vi "Test Driver Message Loop.vi"(8 "error in (no error)":errorcluster) -> (0 "error out":errorcluster)   [LabVIEW 2020, in "Test Driver.lvlib"]
doc: "Message loop for handling messages pertaining to the acquisition of data from the hardware."
uses:
  Test Driver.lvlib
  support/PCT FGV CMD.ctl
  Acquisition State.ctl
  Test Driver Configuration.ctl
  support/Message Queue/Message Cluster.ctl
  System Preset.ctl
  Test Type.ctl
  Popup/Popup Dialog States.ctl
  Motion/AM Configuration.ctl
  support/Message Queue/Enqueue Message (Single).vi
  support/REF Single  Name to ref convert.vi
  <vilib>/Utility/error.llb/Error Cluster From Error Code.vi
  <vilib>/ErrorRing/Error Ring.xnode
  support/Message Queue/Message Queue.lvlib
  Popup/Popup Dialog.lvlib
  Motion/Motion.lvlib
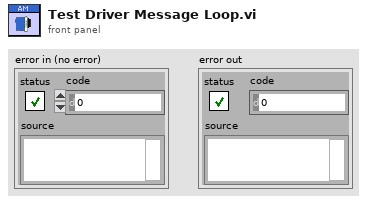
[diagram p1: front panel]
types:
  T1 = typedef "PCT FGV CMD.ctl" = enum16{"INIT", "GET", "SET"}
  T2 = typedef "PCT Data REFs.ctl" = cluster{"PLC AI Notifier":refnum<notifier>, "PS Data Queue":refnum<queue>, "BTN Queue":refnum<queue>, "PLC DI notifier":refnum<notifier>, "Timer notifier":refnum<notifier>, "DMM PS":refnum<notifier>, "DMM Gages":refnum<notifier>, "XYZ notifier":refnum<notifier>, "Test Notifier":refnum<notifier>, "Scanner notifier":refnum<notifier>, "OPC Notifier":refnum<notifier>, "HIDEN queue":refnum<queue>}
  T3 = typedef "Message Queue.lvlib/All Message Queues.ctl" = cluster{"UI":refnum<queue>, "Logging":refnum<queue>, "LOG":refnum<queue>, "ALARM":refnum<queue>, "Test":refnum<queue>, "Answer":refnum<queue>, "PLC":refnum<queue>, "DB":refnum<queue>, "Report":refnum<queue>, "OPC":refnum<queue>, "Procedure":refnum<queue>, "PalmSens":refnum<queue>, "SYS 7000 Reader":refnum<queue>, "SWITCH":refnum<queue>, "MOTOR":refnum<queue>, "MOTION":refnum<queue>, "HIDEN":refnum<queue>, "VALVE":refnum<queue>, "MFC":refnum<queue>, "PUMP IN":refnum<queue>, "PUMP OUT":refnum<queue>}
  T4 = typedef "Test Driver.lvlib/Test Driver Configuration.ctl" = cluster{"current Step":i32, "Wait":dbl, "Next Step":string, "Writer Queue":refnum<queue>, "Reset":bool, "SEQ Time":i32, "General Reset":bool, "Cycles":i32, "Status":bool[], "Ready":bool[], "Backward":bool, "Current SP":dbl[], "System Preset":T5, "Test Type":T6, "Sample Count":i32, "Local Queues":cluster{"Cycles queue":refnum<queue>, "Step queue":refnum<queue>, "RES Queue":refnum<queue>, "Clean queue":refnum<queue>, "PS Scan queue":refnum<queue>}, "current Clean":i32, "PS Measure Plan":u16[]}
  T5 = typedef "System Preset.ctl" = cluster{"Test Configuration":cluster{"Cycles":i32, "Z Up":dbl, "SP List":dbl[][], "Operator":string, "Point Delay":i32, "Z Up 2":dbl, "Cleaning In":dbl, "Cleaning Out":dbl, "Cleaning Cycles":i32}, "Test_Start_date":string}
  T6 = typedef "Test Driver.lvlib/Test Type.ctl" = enum16{"Calibration", "Test"}
  T7 = typedef "Test Driver.lvlib/Acquisition State.ctl" = enum16{"Idle", "Initialized"}
  T8 = typedef "Popup Dialog.lvlib/Popup Dialog States.ctl" = enum32{"Complete", "Failed", "Preparing", "Stopping", "Error", "Saved", "Saving", "Closing"}
  T9 = cluster{"Writer Queue":refnum<queue>, "Timeout":dbl[], "Status":bool[]}
  T10 = typedef "Motion.lvlib/AM Configuration.ctl" = cluster{"Wait":dbl, "Next Step":string, "Writer Queue":refnum<queue>, "Reset":bool, "Target":dbl[]}
  T11 = typedef "Message Queue.lvlib/Message Cluster.ctl" = cluster{"Message":string, "Message Data":variant}
  T12 = typedef "MeasurementResults.ctl" = T13[]
  T13 = typedef "LiveCurveResult.ctl" = cluster{"X Label":string, "Y Label":string, "Name":string, "Index":i16, "Curve Values":cluster{"Values":cluster{"X Value":dbl, "Y Value":dbl}[], "Index":i16}}
  T14 = cluster{"whole match":string, "Results":T12, "Measurements":dbl[]}
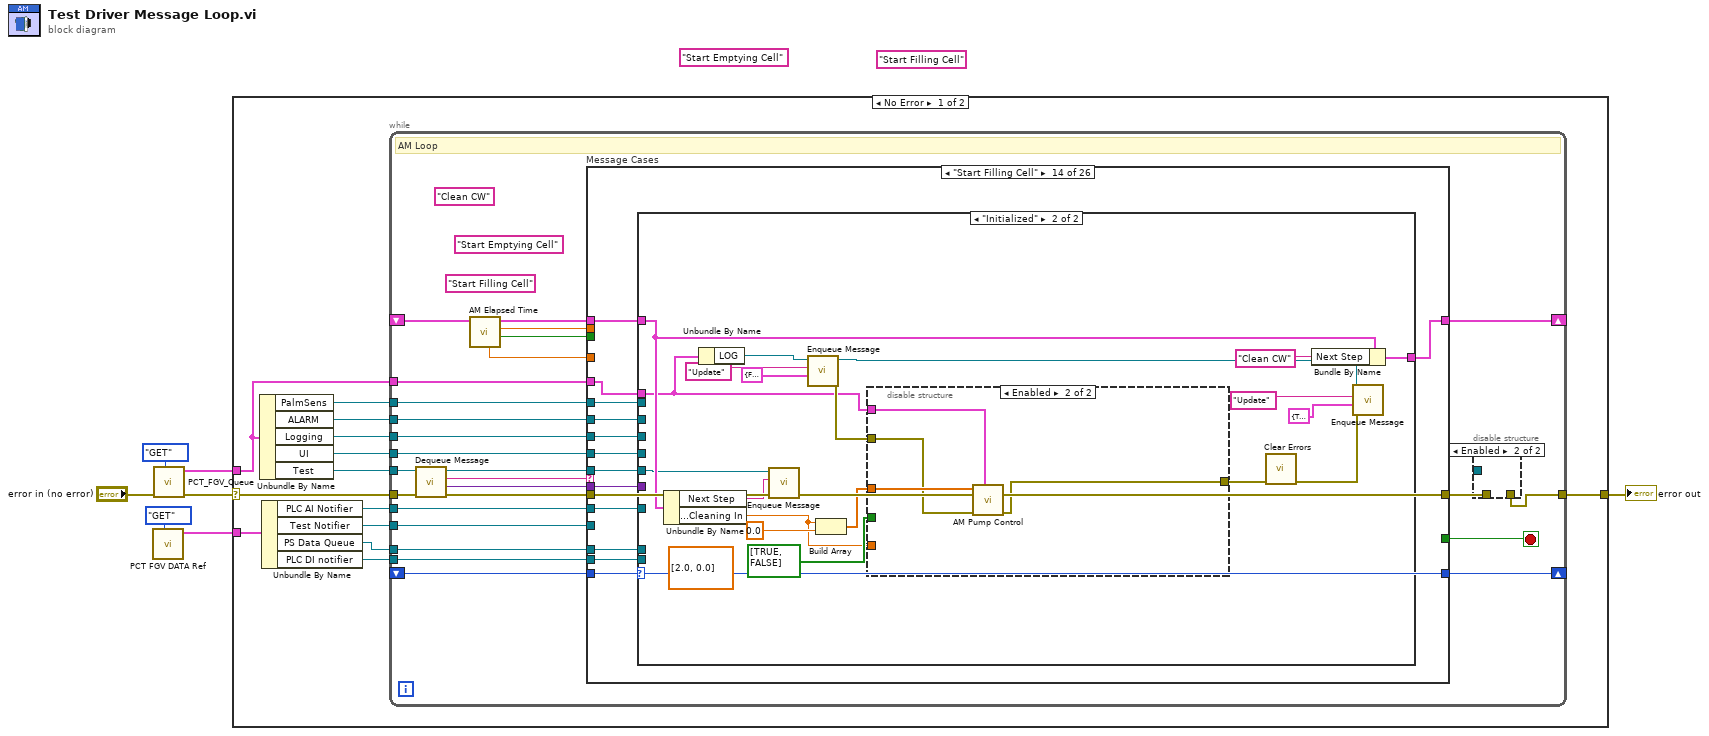
[diagram p0: block diagram]
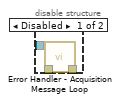
[diagram p2: hidden frame]
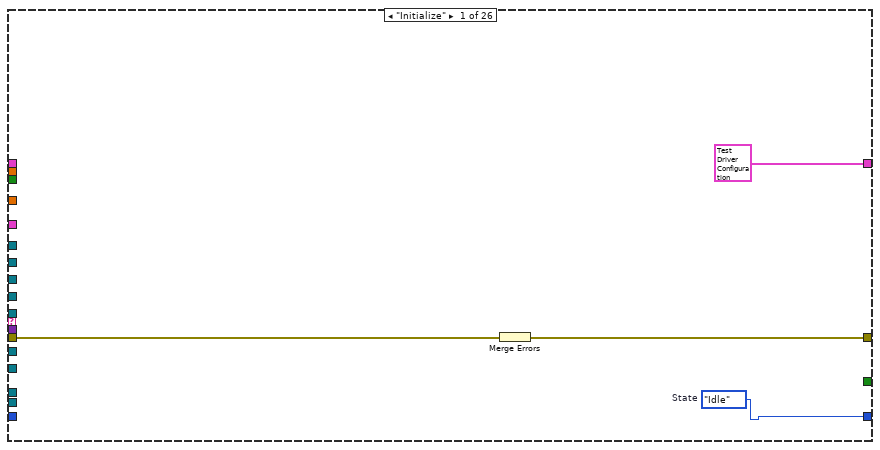
[diagram p3: hidden frame]
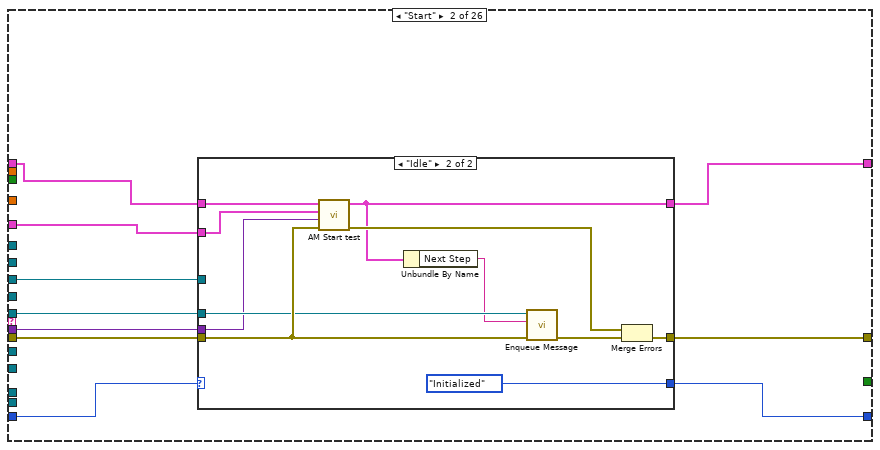
[diagram p4: hidden frame]
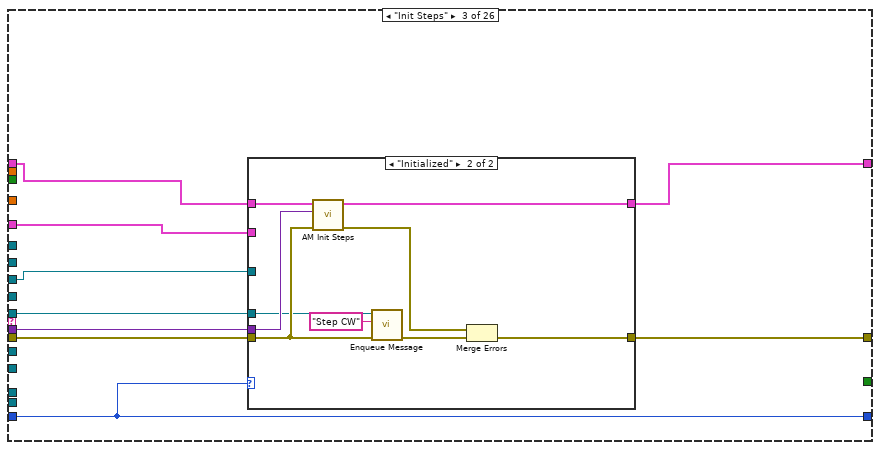
[diagram p6: hidden frame]
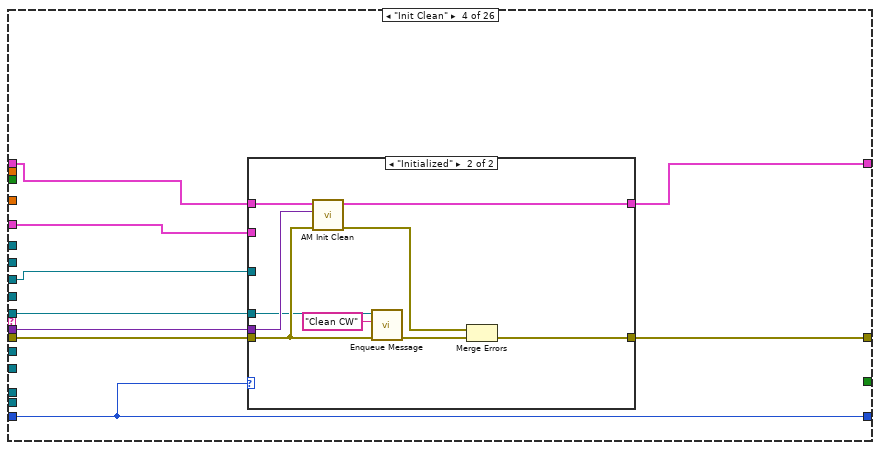
[diagram p8: hidden frame]
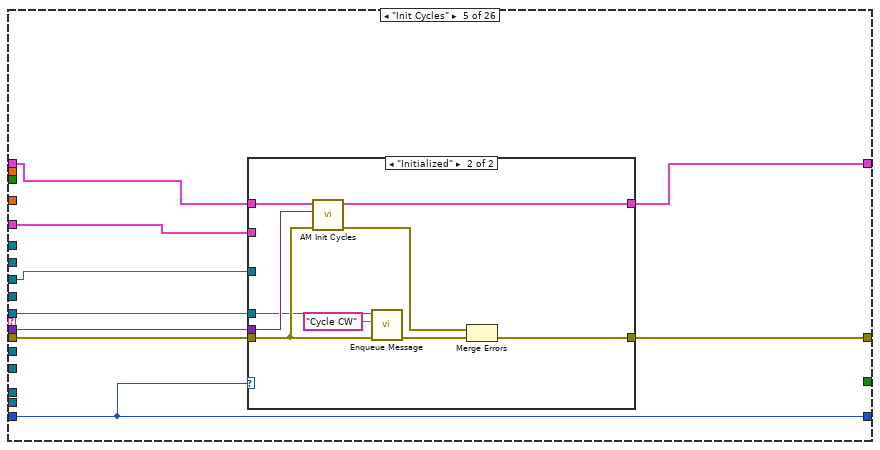
[diagram p10: hidden frame]
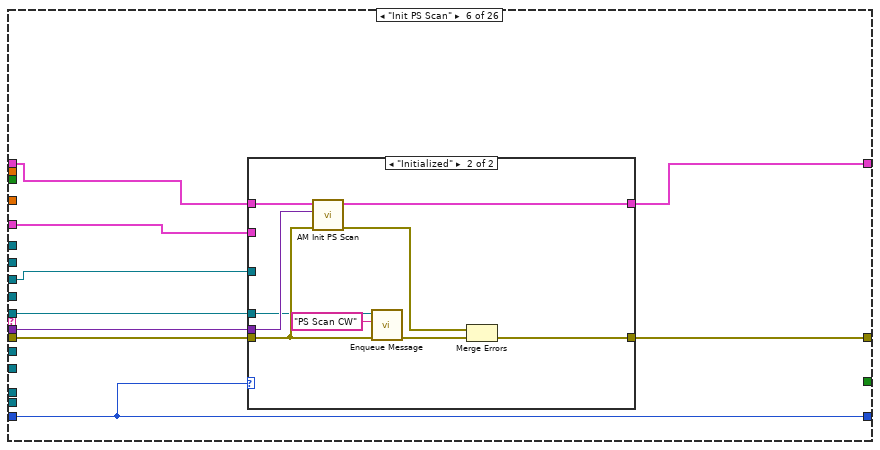
[diagram p12: hidden frame]
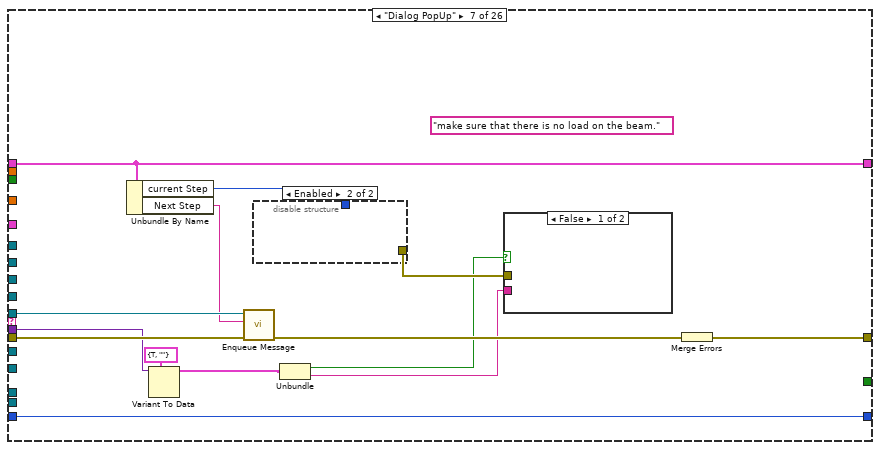
[diagram p14: hidden frame]
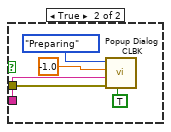
[diagram p15: hidden frame]
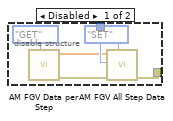
[diagram p16: hidden frame]
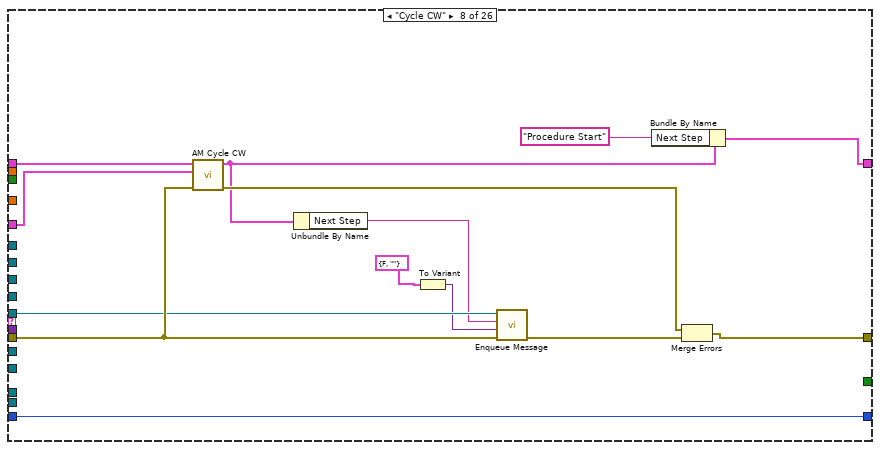
[diagram p17: hidden frame]
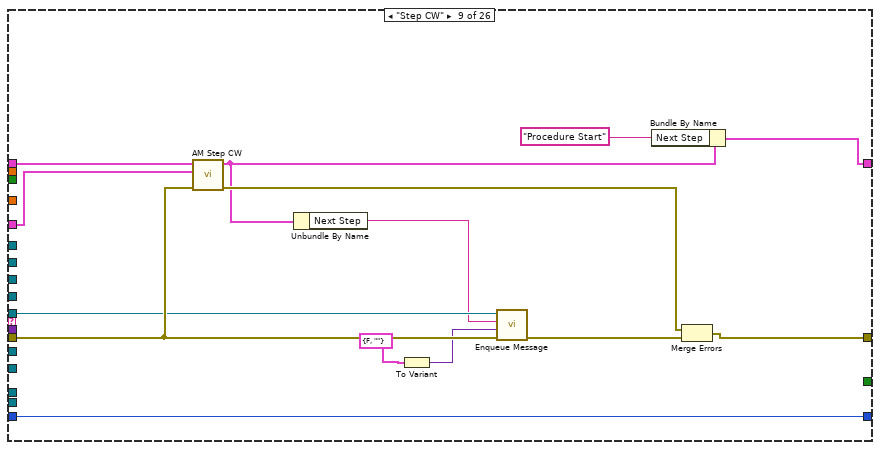
[diagram p18: hidden frame]
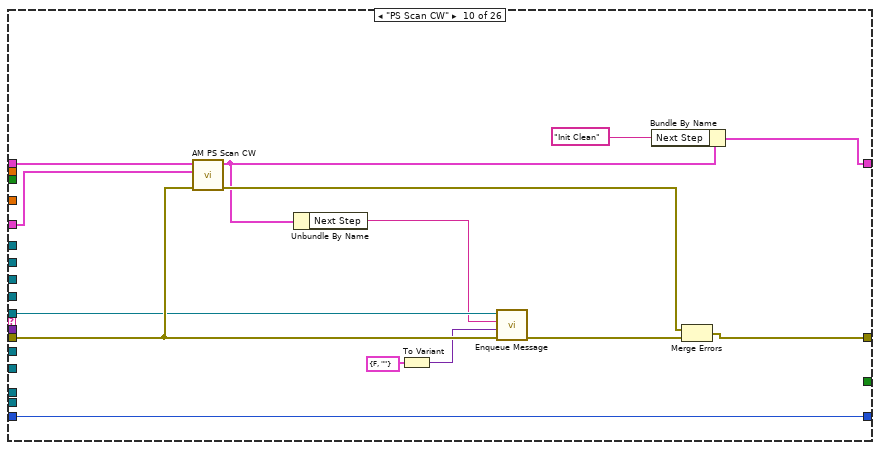
[diagram p19: hidden frame]
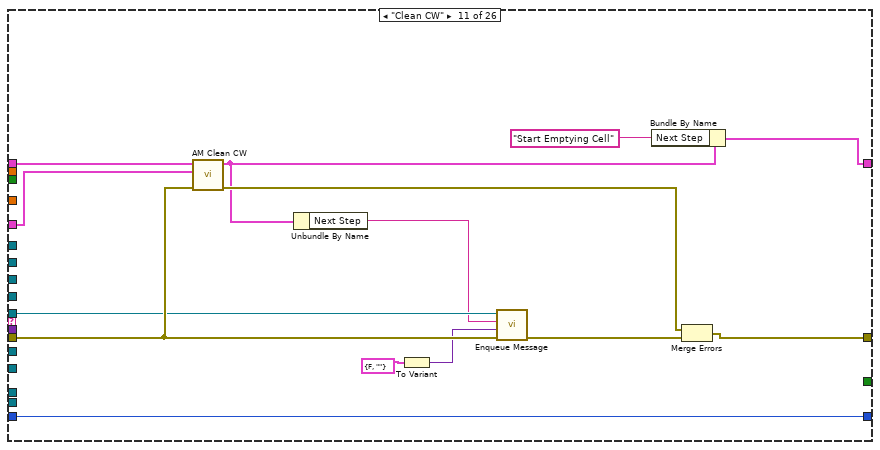
[diagram p20: hidden frame]
diagram:
  (unwired) "Start Filling Cell"
  (unwired) "Start Emptying Cell"
  n1 = call "PCT FGV DATA Ref.vi"("CMD"=PCT_FGV_CMD."GET") -> ("Data REF"=w1:T2)  [unwired: 9 in, 1 out]
  n2 = call "PCT_FGV_Queue.vi"("CMD"=PCT_FGV_CMD."GET", "error in (no error)"="error in (no error)") -> ("error out"=w4:errorcluster, "Message Queues out"=w3:T3)  [unwired: 8 in]
  n3 = case shown="No Error" w4 {
    selector: w4 -> [w18 w653]
    tunnel: w3 -> [w16 _]
    tunnel: [w19 w653] -> w7
    tunnel: w1 -> [w15 _]
    frame No Error {
      n4 = Unbundle By Name(w16) -> ("PalmSens"=w10:refnum<queue>, "ALARM"=w12:refnum<queue>, "Logging"=w13:refnum<queue>, "UI"=w17:refnum<queue>, "Test"=w20:refnum<queue>)
      n5 = Unbundle By Name(w15) -> ("PLC AI Notifier"=w9:refnum<notifier>, "Test Notifier"=w14:refnum<notifier>, "PS Data Queue"=w11:refnum<queue>, "PLC DI notifier"=w8:refnum<notifier>)
      n6 = while {
        tunnel: w20 -> [w39]
        shift-right: [w45] -> _
        shift-left: _ -> [w46]
        tunnel: w17 -> [w33]
        shift-right: [w37] -> _
        shift-left: _ -> [w38]
        tunnel: w16 -> [w29]
        tunnel: w18 -> [w43]
        tunnel: [w36] -> w19
        tunnel: w14 -> [w27]
        tunnel: w13 -> [w26]
        tunnel: w12 -> [w25]
        tunnel: w11 -> [w24]
        tunnel: w10 -> [w23]
        tunnel: w9 -> [w22]
        tunnel: w8 -> [w21]
        stop <- w44 stop-if-true
        (unwired) "Clean CW" ("Message")
        (unwired) "Start Emptying Cell"
        (unwired) "Start Filling Cell" ("Message")
        # "AM Loop"
        n7 = call "Dequeue Message.vi"("error in (no error)"=w43, "Message Queue"=w39) -> ("error out"=w42:errorcluster, "Message Data"=w40:variant, "Message"=w41:string, "dup Message Queue"=w34:refnum<queue>)  [unwired: 6 in]
        n8 = call "AM Elapsed Time.vi"("AM Refs in"=w46) -> ("Time has Elapsed"=w31:bool, "Start Elapsed Time"=w28:dbl, "AM Refs out"=w32:T4, "Elapsed Time (s)"=w30:dbl)  [unwired: 7 in]
        n9 = case "Message Cases" shown="\"Start Filling Cell\"" w41 {
          selector: w41 -> [_ _ _ _ _ _ _ _ _ _ _ w240 _ _ _ _ _ _ _ _ _ _ _ _ _ w642]
          tunnel: w34 -> [_ w60 w83 w103 w123 w143 w168 w190 w204 w218 w232 w247 w263 w319 w377 w436 w481 _ w574 w603 w608 w612 _ _ w636 _]
          tunnel: w42 -> [w52 w61 w84 w104 w124 w144 w169 w191 w205 w219 w233 w248 w265 w321 w379 w438 w500 w537 w575 w604 w609 w616 w624 w628 w638 _]
          tunnel: [w53 w63 w86 w106 w126 w146 w166 w193 w207 w221 w235 w250 w265 w321 w379 w438 w500 w537 w575 w604 w609 w615 w623 w634 w640 w643] -> w35
          tunnel: w32 -> [_ w62 w85 w105 w125 w145 w167 w195 w209 w223 w237 w246 w260 w316 w374 w433 w493 w533 w551 w590 w610 w617 w621 w630 w639 w645]
          tunnel: [T4 {"current Step"=0, "Wait"=0.0, "Next Step"="", "Writer Queue"=refnum, "Reset"=FALSE, "SEQ Time"=0, "General Reset"=FALSE, "Cycles"=0, "Status"=[], "Ready"=[], "Backward"=FALSE, "Current SP"=[], "System Preset"={"Test Configuration"={"Cycles"=0, "Z Up"=0.0, "SP List"=[], "Operator"="", "Point Delay"=0, "Z Up 2"=0.0, "Cleaning In"=0.0, "Cleaning Out"=0.0, "Cleaning Cycles"=0}, "Test_Start_date"=""}, "Test Type"=enum."Calibration", "Sample Count"=0, "Local Queues"={"Cycles queue"=refnum, "Step queue"=refnum, "RES Queue"=refnum, "Clean queue"=refnum, "PS Scan queue"=refnum}, "current Clean"=0, "PS Measure Plan"=[]} ("Data Cluster") w59 w82 w102 w122 w142 w167 w186 w200 w214 w228 w242 w264 w320 w378 w437 w499 w536 w571 w599 w610 w618 w621 w629 w639 w645] -> w45
          tunnel: [_ _ _ _ _ _ _ _ _ _ _ _ _ _ _ _ _ _ _ _ _ _ _ _ TRUE _] -> w44
          tunnel: w40 -> [_ w56 w81 w101 w121 w141 w162 _ _ _ _ w239 w261 w317 w375 w434 _ _ _ _ _ w614 w622 w633 _ _]
          tunnel: w33 -> [_ _ _ _ _ _ _ _ _ _ _ _ w258 w314 w372 w431 _ _ _ _ _ _ _ _ _ _]
          tunnel: w38 -> [_ w57 w79 w99 w119 w139 w171 w196 w210 w224 w238 w251 w252 w308 w366 w425 w501 w538 _ _ _ w619 w625 w627 _ w644]
          tunnel: [w51 w58 w79 w99 w119 w139 w171 w196 w210 w224 w238 w251 w252 w308 w366 w425 w501 w538 Acquisition_State."Idle" ("Acquisition State") Acquisition_State."Idle" ("Acquisition State") Acquisition_State."Idle" ("Acquisition State") w619 w625 w627 Acquisition_State."Idle" ("Acquisition State") w644] -> w37
          tunnel: w31 -> [_ _ _ _ _ _ _ _ _ _ _ w241 _ _ _ _ _ _ _ _ _ _ _ _ _ _]
          tunnel: w30 -> [_ _ _ _ _ _ _ _ _ _ _ _ _ _ _ _ _ _ _ _ _ _ _ _ _ _]
          tunnel: w29 -> [_ w55 w80 w100 w120 w140 _ w194 w208 w222 w236 _ w262 w318 w376 w435 w491 w534 w560 w591 _ w613 _ _ _ _]
          tunnel: w28 -> [_ _ _ _ _ _ _ _ _ _ _ _ _ _ _ _ _ _ _ _ _ _ _ _ _ _]
          tunnel: w27 -> [_ _ _ _ _ _ _ _ _ _ _ _ _ _ _ _ _ w532 _ _ _ _ _ _ _ _]
          tunnel: w26 -> [_ w54 w78 w98 w118 w138 _ _ _ _ _ _ w255 w311 w369 w428 _ _ _ w582 _ _ _ _ _ _]
          tunnel: w25 -> [_ _ _ _ _ _ _ _ _ _ _ _ w259 w315 w373 w432 _ _ _ _ _ _ _ _ _ _]
          tunnel: w24 -> [_ _ _ _ _ _ _ _ _ _ _ _ w257 w313 w371 w430 _ _ _ _ _ _ _ _ _ _]
          tunnel: w23 -> [_ _ _ _ _ _ _ _ _ _ _ _ w256 w312 w370 w429 _ _ _ _ _ _ _ _ _ _]
          tunnel: w22 -> [_ _ _ _ _ _ _ _ _ _ _ _ w254 w310 w368 w427 _ _ _ _ _ _ _ _ _ _]
          tunnel: w21 -> [_ _ _ _ _ _ _ _ _ _ _ _ w253 w309 w367 w426 _ _ _ _ _ _ _ _ _ _]
          frame "Initialize" {
            w51 = Acquisition_State."Idle"  # State
            # "Initialize  - Initialize is currently a no-op.  The hardware initialization takes place in the 'Start' message."
            n10 = Merge Errors(w52) -> (w53:errorcluster)
          }
          frame "Start" {
            # "Start - Configure and start the acquisition."
            n11 = case shown="\"Idle\"" w57 {
              selector: w57 -> [w64 _]
              tunnel: [w65 w77] -> w63
              tunnel: w62 -> [w66 w76]
              tunnel: w61 -> [w65 w73]
              tunnel: w60 -> [_ w71]
              tunnel: [w66 w68] -> w59
              tunnel: [w64 Acquisition_State."Initialized" ("Acquisition State")] -> w58
              tunnel: w56 -> [_ w69]
              tunnel: w55 -> [_ w70]
              tunnel: w54 -> [_ _]
              frame "Initialized" {
                # "The system is already acquiring. Ignore the \"Start\" message."
              }
              frame "Idle" {
                # "If the system is idle, start the acquisition."
                n12 = call "AM Start test.vi"("error in (no error)"=w73, "Variant"=w69, "Message Queues in"=w70, "Hardware Resources in"=w76) -> ("error out"=w75:errorcluster, "Hardware Resources out"=w68:T4)  [unwired: 6 in]
                n13 = Unbundle By Name(w68) -> ("Next Step"=w67:string)
                n14 = call-poly "Enqueue Message.vi"("error in (no error)"=w73, "Message"=w67, "Message Queue"=w71) -> ("error out"=w72:errorcluster)  [unwired: 7 in, 1 out]
                n15 = Merge Errors(w75, w72) -> (w77:errorcluster)
              }
            }
          }
          frame "Init Steps" {
            # "Start - Configure and start the acquisition."
            n16 = case shown="\"Initialized\"" w79 {
              tunnel: [w87 w97] -> w86
              tunnel: w85 -> [w88 w96]
              tunnel: w84 -> [w87 w93]
              tunnel: w83 -> [_ w91]
              tunnel: [w88 w89] -> w82
              tunnel: w81 -> [_ w94]
              tunnel: w80 -> [_ _]
              tunnel: w78 -> [_ _]
              frame "Idle" {
                # "The system is already acquiring. Ignore the \"Start\" message."
              }
              frame "Initialized" {
                # "If the system is idle, start the acquisition."
                n17 = call "AM Init Steps.vi"("error in (no error)"=w93, "Message Data"=w94, "Hardware Resources in"=w96) -> ("error out"=w95:errorcluster, "Hardware Resources out"=w89:T4)  [unwired: 7 in]
                n18 = call-poly "Enqueue Message.vi"("error in (no error)"=w93, "Message"="Step CW", "Message Queue"=w91) -> ("error out"=w92:errorcluster)  [unwired: 7 in, 1 out]
                n19 = Merge Errors(w95, w92) -> (w97:errorcluster)
              }
            }
          }
          frame "Init Clean" {
            # "Start - Configure and start the acquisition."
            n20 = case shown="\"Initialized\"" w99 {
              tunnel: [w107 w117] -> w106
              tunnel: w105 -> [w108 w116]
              tunnel: w104 -> [w107 w113]
              tunnel: w103 -> [_ w111]
              tunnel: [w108 w109] -> w102
              tunnel: w101 -> [_ w114]
              tunnel: w100 -> [_ _]
              tunnel: w98 -> [_ _]
              frame "Idle" {
                # "The system is already acquiring. Ignore the \"Start\" message."
              }
              frame "Initialized" {
                # "If the system is idle, start the acquisition."
                n21 = call "AM Init Clean.vi"("error in (no error)"=w113, "Message Data"=w114, "Hardware Resources in"=w116) -> ("error out"=w115:errorcluster, "Hardware Resources out"=w109:T4)  [unwired: 7 in]
                n22 = call-poly "Enqueue Message.vi"("error in (no error)"=w113, "Message"="Clean CW", "Message Queue"=w111) -> ("error out"=w112:errorcluster)  [unwired: 7 in, 1 out]
                n23 = Merge Errors(w115, w112) -> (w117:errorcluster)
              }
            }
          }
          frame "Init Cycles" {
            # "Start - Configure and start the acquisition."
            n24 = case shown="\"Initialized\"" w119 {
              tunnel: [w127 w137] -> w126
              tunnel: w125 -> [w128 w136]
              tunnel: w124 -> [w127 w133]
              tunnel: w123 -> [_ w131]
              tunnel: [w128 w129] -> w122
              tunnel: w121 -> [_ w134]
              tunnel: w120 -> [_ _]
              tunnel: w118 -> [_ _]
              frame "Idle" {
                # "The system is already acquiring. Ignore the \"Start\" message."
              }
              frame "Initialized" {
                # "If the system is idle, start the acquisition."
                n25 = call "AM Init Cycles.vi"("error in (no error)"=w133, "Message Data"=w134, "Hardware Resources in"=w136) -> ("error out"=w135:errorcluster, "Hardware Resources out"=w129:T4)  [unwired: 7 in]
                n26 = call-poly "Enqueue Message.vi"("error in (no error)"=w133, "Message"="Cycle CW", "Message Queue"=w131) -> ("error out"=w132:errorcluster)  [unwired: 7 in, 1 out]
                n27 = Merge Errors(w135, w132) -> (w137:errorcluster)
              }
            }
          }
          frame "Init PS Scan" {
            # "Start - Configure and start the acquisition."
            n28 = case shown="\"Initialized\"" w139 {
              tunnel: [w147 w157] -> w146
              tunnel: w145 -> [w148 w156]
              tunnel: w144 -> [w147 w153]
              tunnel: w143 -> [_ w151]
              tunnel: [w148 w149] -> w142
              tunnel: w141 -> [_ w154]
              tunnel: w140 -> [_ _]
              tunnel: w138 -> [_ _]
              frame "Idle" {
                # "The system is already acquiring. Ignore the \"Start\" message."
              }
              frame "Initialized" {
                # "If the system is idle, start the acquisition."
                n29 = call "AM Init PS Scan.vi"("error in (no error)"=w153, "Message Data"=w154, "Hardware Resources in"=w156) -> ("error out"=w155:errorcluster, "Hardware Resources out"=w149:T4)  [unwired: 7 in]
                n30 = call-poly "Enqueue Message.vi"("error in (no error)"=w153, "Message"="PS Scan CW", "Message Queue"=w151) -> ("error out"=w152:errorcluster)  [unwired: 7 in, 1 out]
                n31 = Merge Errors(w155, w152) -> (w157:errorcluster)
              }
            }
          }
          frame "Dialog PopUp" {
            (unwired) "make sure that there is no load on the beam." ("String")
            # "Start - Configure and start the acquisition."
            n32 = Unbundle By Name(w167) -> ("current Step"=w165:i32, "Next Step"=w164:string)
            n33 = Variant To Data(type=cluster{"Show":bool, "Message":string} {"Show"=TRUE, "Message"=""}, Variant=w162) -> (data=w160:cluster{"Show":bool, "Message":string})  [unwired: 1 in, 1 out]
            n34 = call-poly "Enqueue Message.vi"("error in (no error)"=w169, "Message"=w164, "Message Queue"=w168) -> ("error out"=w170:errorcluster)  [unwired: 7 in, 1 out]
            n35 = disable-structure shown="Enabled" {
              disable-tunnel: w165 -> [w182 _]
              disable-tunnel: [w178 _] -> w163
              frame Disabled {
                n36 = call "AM FGV Data per Step.vi"("CMD"=PCT_FGV_CMD."GET") -> ("error out"=w179:errorcluster, "All Data out"=w177:dbl[])  [unwired: 9 in]
                n37 = call "AM FGV All Step Data.vi"("CMD"=PCT_FGV_CMD."SET", "error in (no error)"=w179, "current Step"=w182, "Proc Data in"=w177) -> ("error out"=w178:errorcluster)  [unwired: 6 in, 1 out]
              }
              frame Enabled {
              }
            }
            n38 = Unbundle(w160) -> ("Show"=w159:bool, "Message"=w158:string)
            n39 = case shown="False" w159 {
              tunnel: w163 -> [_ w175]
              tunnel: w158 -> [_ w173]
              frame False {
              }
              frame True {
                n40 = call "Popup Dialog CLBK.vi"("show"=TRUE, "error in"=w175, "String"=w173, "Delay (5sec)"=-1.0, "Tab Control"=Popup_Dialog_States."Preparing") -> ()  [unwired: 4 in, 3 out]
              }
            }
            n41 = Merge Errors(w170) -> (w166:errorcluster)
          }
          frame "Cycle CW" {
            # "Start - Configure and start the acquisition."
            n42 = call "AM Cycle CW.vi"("error in (no error)"=w191, "Message Queues in"=w194, "Data Cluster"=w195) -> ("error out"=w188:errorcluster, "Data Cluster out"=w187:T4)  [unwired: 7 in]
            n43 = Unbundle By Name(w187) -> ("Next Step"=w189:string)
            n44 = To Variant(anything=cluster{"Show":bool, "Message":string} {"Show"=FALSE, "Message"=""}) -> (Variant=w183:variant)
            n45 = call-poly "Enqueue Message.vi"("error in (no error)"=w191, "Message Data"=w183, "Message"=w189, "Message Queue"=w190) -> ("error out"=w192:errorcluster)  [unwired: 6 in, 1 out]
            n46 = Bundle By Name(cluster=w187, "Next Step"="Procedure Start" ("Message")) -> (w186:T4)
            n47 = Merge Errors(w188, w192) -> (w193:errorcluster)
          }
          frame "Step CW" {
            # "Start - Configure and start the acquisition."
            n48 = call "AM Step CW.vi"("error in (no error)"=w205, "Message Queues in"=w208, "Data Cluster"=w209) -> ("error out"=w202:errorcluster, "Data Cluster out"=w201:T4)  [unwired: 7 in]
            n49 = Unbundle By Name(w201) -> ("Next Step"=w203:string)
            n50 = To Variant(anything=cluster{"Show":bool, "Message":string} {"Show"=FALSE, "Message"=""}) -> (Variant=w197:variant)
            n51 = call-poly "Enqueue Message.vi"("error in (no error)"=w205, "Message Data"=w197, "Message"=w203, "Message Queue"=w204) -> ("error out"=w206:errorcluster)  [unwired: 6 in, 1 out]
            n52 = Bundle By Name(cluster=w201, "Next Step"="Procedure Start" ("Message")) -> (w200:T4)
            n53 = Merge Errors(w202, w206) -> (w207:errorcluster)
          }
          frame "PS Scan CW" {
            # "Start - Configure and start the acquisition."
            n54 = call "AM PS Scan CW.vi"("error in (no error)"=w219, "Message Queues in"=w222, "Data Cluster"=w223) -> ("error out"=w216:errorcluster, "Data Cluster out"=w215:T4)  [unwired: 7 in]
            n55 = Unbundle By Name(w215) -> ("Next Step"=w217:string)
            n56 = To Variant(anything=cluster{"Show":bool, "Message":string} {"Show"=FALSE, "Message"=""}) -> (Variant=w211:variant)
            n57 = call-poly "Enqueue Message.vi"("error in (no error)"=w219, "Message Data"=w211, "Message"=w217, "Message Queue"=w218) -> ("error out"=w220:errorcluster)  [unwired: 6 in, 1 out]
            n58 = Bundle By Name(cluster=w215, "Next Step"="Init Clean" ("Message")) -> (w214:T4)
            n59 = Merge Errors(w216, w220) -> (w221:errorcluster)
          }
          frame "Clean CW" {
            # "Start - Configure and start the acquisition."
            n60 = call "AM Clean CW.vi"("error in (no error)"=w233, "Message Queues in"=w236, "Data Cluster"=w237) -> ("error out"=w230:errorcluster, "Data Cluster out"=w229:T4)  [unwired: 7 in]
            n61 = Unbundle By Name(w229) -> ("Next Step"=w231:string)
            n62 = To Variant(anything=cluster{"Show":bool, "Message":string} {"Show"=FALSE, "Message"=""}) -> (Variant=w226:variant)
            n63 = call-poly "Enqueue Message.vi"("error in (no error)"=w233, "Message Data"=w226, "Message"=w231, "Message Queue"=w232) -> ("error out"=w234:errorcluster)  [unwired: 6 in, 1 out]
            n64 = Bundle By Name(cluster=w229, "Next Step"="Start Emptying Cell") -> (w228:T4)
            n65 = Merge Errors(w230, w234) -> (w235:errorcluster)
          }
          frame "Wait" {
            # "Start - Configure and start the acquisition."
            n66 = Unbundle By Name(w246) -> ("Next Step"=w245:string)
            n67 = Wait Until Next ms Multiple(millisecond multiple=u32 200) -> ()  [unwired: 1 out]
            n68 = Select(t=w245, s=w241, f=w240) -> (s? t:f=w244:string)
            n69 = Bundle By Name(cluster=w246, "Reset"=w241) -> (w242:T4)
            n70 = call-poly "Enqueue Message.vi"("error in (no error)"=w248, "Message Data"=w239, "Message"=w244, "Message Queue"=w247) -> ("error out"=w249:errorcluster)  [unwired: 6 in, 1 out]
            n71 = Merge Errors(w249) -> (w250:errorcluster)
          }
          frame "Procedure Response" {
            # "Start - Configure and start the acquisition."
            n72 = case shown="\"Initialized\"" w252 {
              tunnel: [w266 w303] -> w264
              tunnel: w263 -> [_ w301]
              tunnel: w262 -> [_ w293]
              tunnel: w261 -> [_ _]
              tunnel: w260 -> [w266 w292]
              tunnel: w259 -> [_ w291]
              tunnel: w258 -> [_ w282]
              tunnel: w257 -> [_ _]
              tunnel: w256 -> [_ _]
              tunnel: w255 -> [_ _]
              tunnel: w254 -> [_ _]
              tunnel: w253 -> [_ _]
              frame "Idle", Default {
              }
              frame "Initialized" {
                (unwired) "PS Scan"
                w272 = PCT_FGV_CMD."SET" ("CMD")
                n73 = call-poly "Enqueue Message.vi"("Message"="Stop", "Message Queue"=w291) -> ()  [unwired: 8 in, 2 out]
                n74 = Unbundle By Name(w292) -> ("Current SP"=w283:dbl[], "current Step"=w268:i32, "Cycles"=w271:i32)
                n75 = call-poly "Enqueue Message.vi"("Message"="Start Filling Cell", "Message Queue"=w301) -> ()  [unwired: 8 in, 2 out]
                n76 = Build Array (concatenate)(w283, w268) -> (w276:dbl[])
                n77 = for {
                  tunnel: string[] ["X%0.1f ", "Y%0.1f "] ("format string") -> [w307] mode=indexing
                  tunnel: w283 -> [w306] mode=indexing
                  shift-right: [w305] -> w288
                  shift-left: "" -> [w304]
                  n78 = Format Into String(format string=w307, initial string=w304, w306) -> (resulting string=w305:string)  [unwired: 1 in, 1 out]
                }
                n79 = call "FGV Parameters.vi"("CMD"=w272, "input"=w268, "Key"="Step") -> ("error out"=w269:errorcluster)  [unwired: 6 in, 2 out]
                n80 = call "FGV Parameters.vi"("CMD"=w272, "error in (no error)"=w269, "input"=w271, "Key"="Cycle") -> ()  [unwired: 5 in, 3 out]
                n81 = Format Into String(format string="Movement to %s has finished", w288) -> (resulting string=w295:string)  [unwired: 2 in, 1 out]
                n82 = Unbundle By Name(w293) -> ("LOG"=w294:refnum<queue>)
                n83 = Reverse 1D Array(array=w276) -> (reversed array=w274:dbl[])
                n84 = Bundle By Name(cluster=cluster{"Replace":bool, "String":string} {"Replace"=FALSE, "String"="Procedure was started"}, "String"=w295) -> (w296:cluster{"Replace":bool, "String":string})
                n85 = Number To Fractional String(number=w274, precision (6)=i16 1) -> (F-format string=w275:string[])  [unwired: 2 in]
                n86 = call "Bundle CMD Queue Cluster.vi"("Message Data"=w276, "Message"="Update Procedure" ("Type CMD")) -> ("Message Cluster"=w286:T11)  [unwired: 9 in]
                n87 = call "Bundle CMD Queue Cluster.vi"("Message Data"=w275, "Message"="Update RES Table" ("Type CMD")) -> ("Message Cluster"=w280:T11)  [unwired: 9 in]
                n88 = call-poly "Enqueue Message.vi"("Message Data"=w286, "Message"="Update Status" ("Main CMD"), "Message Queue"=w282) -> ("dup Message Queue"=w278:refnum<queue>)  [unwired: 7 in, 1 out]
                n89 = call-poly "Enqueue Message.vi"("Message Data"=w296, "Message"="Update" ("Main CMD"), "Message Queue"=w294) -> ()  [unwired: 7 in, 2 out]
                n90 = Bundle By Name(cluster=w292, "Next Step"="Init PS Scan") -> (w303:T4)
                n91 = call-poly "Enqueue Message.vi"("Priority Message? (F)"=TRUE, "Message Data"=w280, "Message"="Update Status", "Message Queue"=w278) -> ()  [unwired: 6 in, 2 out]
              }
            }
          }
          frame "Start Filling Cell" {
            # "Start - Configure and start the acquisition."
            n92 = case shown="\"Initialized\"" w308 {
              tunnel: [w322 w341] -> w320
              tunnel: w319 -> [_ w336]
              tunnel: w318 -> [_ w323]
              tunnel: w317 -> [_ _]
              tunnel: w316 -> [w322 w338]
              tunnel: w315 -> [_ _]
              tunnel: w314 -> [_ _]
              tunnel: w313 -> [_ _]
              tunnel: w312 -> [_ _]
              tunnel: w311 -> [_ _]
              tunnel: w310 -> [_ _]
              tunnel: w309 -> [_ _]
              frame "Idle", Default {
              }
              frame "Initialized" {
                (unwired) dbl[] [2.0, 0.0] ("Timeout")
                n93 = Unbundle By Name(w338) -> ("Next Step"=w328:string, "System Preset.Test Configuration.Cleaning In"=w324:dbl)
                n94 = Unbundle By Name(w323) -> ("LOG"=w331:refnum<queue>)
                n95 = call-poly "Enqueue Message.vi"("Message"=w328, "Message Queue"=w336) -> ()  [unwired: 8 in, 2 out]
                n96 = call-poly "Enqueue Message.vi"("Message Data"=cluster{"Replace":bool, "String":string} {"Replace"=FALSE, "String"="Cell Filling->START"}, "Message"="Update" ("Main CMD"), "Message Queue"=w331) -> ("error out"=w329:errorcluster, "dup Message Queue"=w330:refnum<queue>)  [unwired: 7 in]
                n97 = Build Array(w324, 0.0 ("Timeout")) -> (w325:dbl[])
                n98 = disable-structure shown="Enabled" {
                  disable-tunnel: w323 -> [w355 w362]
                  disable-tunnel: bool[] [TRUE, FALSE] ("Status") -> [w352 _]
                  disable-tunnel: [w347 w364] -> w335
                  disable-tunnel: w329 -> [w346 w363]
                  disable-tunnel: w325 -> [w344 w365]
                  disable-tunnel: w324 -> [w343 _]
                  frame Disabled {
                    n99 = call "Obtain Message Queue.vi"() -> ("Message Queue"=w351:refnum<queue>)  [unwired: 10 in, 1 out]
                    n100 = Bundle By Name(cluster=T9 {"Writer Queue"=refnum, "Timeout"=[], "Status"=[]}, "Writer Queue"=w351, "Timeout"=w344, "Status"=w352) -> (w353:T9)
                    n101 = call-poly "Enqueue Message.vi"("error in (no error)"=w346, "Message Data"=w353, "Message"="Start", "Message Queue"=w355) -> ("error out"=w350:errorcluster)  [unwired: 6 in, 1 out]
                    n102 = Multiply(x=w343, y=2000.0) -> (x*y=w348:dbl)
                    n103 = for {
                      N: 2 -> [_]
                      tunnel: w348 -> [w358]
                      shift-right: [w357] -> w342
                      shift-left: w351 -> [w361]
                      tunnel: w350 -> [w360]
                      tunnel: [w359] -> w347
                      n104 = Dequeue Element(queue=w361, timeout in ms (-1)=w358, error in (no error)=w360) -> (queue out=w357:refnum<queue>, error out=w359:errorcluster)  [unwired: 2 out]
                    }
                    n105 = Release Queue(queue=w342) -> ()  [unwired: 2 in, 3 out]
                  }
                  frame Enabled {
                    n106 = call "AM Pump Control.vi"("input cluster"=w362, "error in (no error)"=w363, "Times"=w365) -> ("error out"=w364:errorcluster)  [unwired: 8 in]
                  }
                }
                n107 = call <vilib>:"Clear Errors.vi"("error in (no error)"=w335) -> ("error out"=w334:errorcluster)  [unwired: 5 in, 1 out]
                n108 = Bundle By Name(cluster=w338, "Next Step"="Clean CW" ("Message")) -> (w341:T4)
                n109 = call-poly "Enqueue Message.vi"("error in (no error)"=w334, "Message Data"=cluster{"Replace":bool, "String":string} {"Replace"=TRUE, "String"="Cell Filling->DONE"}, "Message"="Update" ("Main CMD"), "Message Queue"=w330) -> ()  [unwired: 6 in, 2 out]
              }
            }
          }
          frame "Start Emptying Cell" {
            # "Start - Configure and start the acquisition."
            n110 = case shown="\"Initialized\"" w366 {
              tunnel: [w380 w399] -> w378
              tunnel: w377 -> [_ w395]
              tunnel: w376 -> [_ w381]
              tunnel: w375 -> [_ _]
              tunnel: w374 -> [w380 w387]
              tunnel: w373 -> [_ _]
              tunnel: w372 -> [_ _]
              tunnel: w371 -> [_ _]
              tunnel: w370 -> [_ _]
              tunnel: w369 -> [_ _]
              tunnel: w368 -> [_ _]
              tunnel: w367 -> [_ _]
              frame "Idle", Default {
              }
              frame "Initialized" {
                (unwired) dbl[] [0.0, 5.0] ("Timeout")
                n111 = Unbundle By Name(w381) -> ("LOG"=w390:refnum<queue>)
                n112 = Unbundle By Name(w387) -> ("Next Step"=w386:string, "System Preset.Test Configuration.Cleaning Out"=w383:dbl)
                n113 = call-poly "Enqueue Message.vi"("Message"=w386, "Message Queue"=w395) -> ()  [unwired: 8 in, 2 out]
                n114 = call-poly "Enqueue Message.vi"("Message Data"=cluster{"Replace":bool, "String":string} {"Replace"=FALSE, "String"="Cell Emptying>START"}, "Message"="Update" ("Main CMD"), "Message Queue"=w390) -> ("error out"=w388:errorcluster, "dup Message Queue"=w389:refnum<queue>)  [unwired: 7 in]
                n115 = Build Array(0.0 ("Timeout"), w383) -> (w382:dbl[])
                n116 = disable-structure shown="Enabled" {
                  disable-tunnel: w381 -> [w414 w422]
                  disable-tunnel: bool[] [FALSE, TRUE] ("Status") -> [w411 _]
                  disable-tunnel: [w405 w423] -> w394
                  disable-tunnel: w388 -> [w404 w421]
                  disable-tunnel: w382 -> [w401 w424]
                  frame Disabled {
                    n117 = call "Obtain Message Queue.vi"() -> ("Message Queue"=w410:refnum<queue>)  [unwired: 10 in, 1 out]
                    n118 = Bundle By Name(cluster=T9 {"Writer Queue"=refnum, "Timeout"=[], "Status"=[]}, "Writer Queue"=w410, "Timeout"=w401, "Status"=w411) -> (w412:T9)
                    n119 = Index Array(array=w401, index=1) -> (element=w408:dbl)
                    n120 = call-poly "Enqueue Message.vi"("error in (no error)"=w404, "Message Data"=w412, "Message"="Start", "Message Queue"=w414) -> ("error out"=w409:errorcluster)  [unwired: 6 in, 1 out]
                    n121 = Multiply(x=w408, y=2000.0) -> (x*y=w406:dbl)
                    n122 = for {
                      N: 2 -> [_]
                      tunnel: w406 -> [w418]
                      shift-right: [w416] -> w400
                      shift-left: w410 -> [w420]
                      tunnel: w409 -> [w419]
                      tunnel: [w417] -> w405
                      n123 = Dequeue Element(queue=w420, timeout in ms (-1)=w418, error in (no error)=w419) -> (queue out=w416:refnum<queue>, error out=w417:errorcluster)  [unwired: 2 out]
                    }
                    n124 = Release Queue(queue=w400) -> ()  [unwired: 2 in, 3 out]
                  }
                  frame Enabled {
                    n125 = call "AM Pump Control.vi"("input cluster"=w422, "error in (no error)"=w421, "Times"=w424) -> ("error out"=w423:errorcluster)  [unwired: 8 in]
                  }
                }
                n126 = call <vilib>:"Clear Errors.vi"("error in (no error)"=w394) -> ("error out"=w393:errorcluster)  [unwired: 5 in, 1 out]
                n127 = Bundle By Name(cluster=w387, "Next Step"="Start Emptying Cell") -> (w399:T4)
                n128 = call-poly "Enqueue Message.vi"("error in (no error)"=w393, "Message Data"=cluster{"Replace":bool, "String":string} {"Replace"=TRUE, "String"="Cell Emptying>DONE"}, "Message"="Update" ("Main CMD"), "Message Queue"=w389) -> ()  [unwired: 6 in, 2 out]
              }
            }
          }
          frame "PS Scan" {
            # "Start - Configure and start the acquisition."
            n129 = case shown="\"Initialized\"" w425 {
              tunnel: [w439 w480] -> w437
              tunnel: w436 -> [_ w478]
              tunnel: w435 -> [_ w475]
              tunnel: w434 -> [_ _]
              tunnel: w433 -> [w439 w474]
              tunnel: w432 -> [_ _]
              tunnel: w431 -> [_ w446]
              tunnel: w430 -> [_ w473]
              tunnel: w429 -> [_ w472]
              tunnel: w428 -> [_ w470]
              tunnel: w427 -> [_ w469]
              tunnel: w426 -> [_ w465]
              frame "Idle", Default {
              }
              frame "Initialized" {
                (unwired) "Start Emptying Cell" ("Message")
                (unwired) "Init Clean"
                w460 = "PS Name Scan" ("Key")
                (unwired) TRUE ("Priority Message? (F)")
                n130 = Unbundle By Name(w475) -> ("LOG"=w456:refnum<queue>)
                n131 = call "FGV Parameters.vi"("CMD"=PCT_FGV_CMD."GET", "Key"=w460) -> ("output"=w461:variant)  [unwired: 7 in, 2 out]
                n132 = Variant To Data(type=w460, Variant=w461) -> (data=w445:string)  [unwired: 1 in, 1 out]
                n133 = call-poly "Enqueue Message.vi"("Message"="PS Scan CW", "Message Queue"=w478) -> ()  [unwired: 8 in, 2 out]
                n134 = call "PS long Name to Short.vi"("String"=w445) -> ("whole match"=w441:string)  [unwired: 10 in]
                n135 = Format Into String(format string="PS->%s->START" ("Message"), w441) -> (resulting string=w451:string)  [unwired: 2 in, 1 out]
                n136 = Bundle By Name(cluster=cluster{"Replace":bool, "String":string} {"Replace"=FALSE, "String"="PS Scanning->START"}, "String"=w451) -> (w452:cluster{"Replace":bool, "String":string})
                n137 = call-poly "Enqueue Message.vi"("Message Data"=w452, "Message"="Update" ("Main CMD"), "Message Queue"=w456) -> ("error out"=w454:errorcluster, "dup Message Queue"=w455:refnum<queue>)  [unwired: 7 in]
                n138 = Send Notification(notification=bool[] [TRUE], notifier=w465, error in (no error)=w454) -> (notifier out=w466:refnum<notifier>, error out=w464:errorcluster)
                n139 = call "Scope Get Trace State Machine.vi"("Type Measurement"=w441, "error in (no error)"=w464, "Data Queue"=w473, "Queue in"=w472) -> ("error out"=w463:errorcluster, "Measurements"=w440:dbl[], "Results"=w442:T12)  [unwired: 5 in]
                n140 = Send Notification(notification=bool[] [FALSE], notifier=w466, error in (no error)=w463) -> ()  [unwired: 2 out]
                n141 = Bundle("whole match"=w441, "Results"=w442, "Measurements"=w440) -> (w443:T14)  [unwired: 1 in]
                n142 = Send Notification(notification=w440, notifier=w469) -> (error out=w444:errorcluster)  [unwired: 1 in, 1 out]
                n143 = call-poly "Enqueue Message.vi"("Message Data"=w445, "Message"="PS Measure Type Update", "Message Queue"=w446) -> ()  [unwired: 7 in, 2 out]
                n144 = call-poly "Enqueue Message.vi"("Message Data"=w443, "Message"="Log", "Message Queue"=w470) -> ()  [unwired: 7 in, 2 out]
                n145 = Format Into String(format string="PS->%s->DONE" ("Message"), w441) -> (resulting string=w448:string)  [unwired: 2 in, 1 out]
                n146 = Bundle By Name(cluster=cluster{"Replace":bool, "String":string} {"Replace"=TRUE, "String"="PS Scanning->DONE"}, "String"=w448) -> (w449:cluster{"Replace":bool, "String":string})
                n147 = call-poly "Enqueue Message.vi"("error in (no error)"=w444, "Message Data"=w449, "Message"="Update" ("Main CMD"), "Message Queue"=w455) -> ()  [unwired: 6 in, 2 out]
                n148 = Bundle By Name(cluster=w474, "Next Step"="PS Scan CW") -> (w480:T4)
              }
            }
          }
          frame "Procedure Pause" {
            # "Start - Configure and start the acquisition."
            n149 = Flush Queue(queue=w481) -> ()  [unwired: 1 in, 3 out]
            n150 = Unbundle By Name(w491) -> ("MOTION"=w490:refnum<queue>)
            n151 = Unbundle By Name(w493) -> ("Local Queues.Step queue"=w488:refnum<queue>, "Current SP"=w487:dbl[])
            n152 = Enqueue Element At Opposite End(queue=w488, element=w487) -> ()  [unwired: 2 in, 3 out]
            n153 = for {
              tunnel: string[] ["X%0.1f ", "Y%0.1f "] ("format string") -> [w505] mode=indexing
              tunnel: w487 -> [w504] mode=indexing
              shift-right: [w503] -> w485
              shift-left: "" -> [w502]
              n154 = Format Into String(format string=w505, initial string=w502, w504) -> (resulting string=w503:string)  [unwired: 1 in, 1 out]
            }
            n155 = call-poly "Enqueue Message.vi"("Priority Message? (F)"=TRUE, "Message"="Procedure Pause" ("Main CMD"), "Message Queue"=w490) -> ()  [unwired: 7 in, 2 out]
            n156 = Unbundle By Name(w491) -> ("LOG"=w494:refnum<queue>)
            n157 = Format Into String(format string="Movement to %s has paused", w485) -> (resulting string=w483:string)  [unwired: 2 in, 1 out]
            n158 = Bundle By Name(cluster=cluster{"Replace":bool, "String":string} {"Replace"=FALSE, "String"="Procedure was started"}, "String"=w483) -> (w495:cluster{"Replace":bool, "String":string})
            n159 = call-poly "Enqueue Message.vi"("Message Data"=w495, "Message"="Update" ("Main CMD"), "Message Queue"=w494) -> ()  [unwired: 7 in, 2 out]
            n160 = Bundle By Name(cluster=w493, "Next Step"="Cycle CW") -> (w499:T4)
          }
          frame "Procedure Start" {
            (unwired) 0 ("Current SP")
            # "Start - Configure and start the acquisition."
            n161 = Unbundle By Name(w534) -> ("ALARM"=w522:refnum<queue>, "MOTION"=w531:refnum<queue>, "LOG"=w528:refnum<queue>)
            n162 = Unbundle By Name(w533) -> ("System Preset.Test Configuration.Point Delay"=w514:i32, "Current SP"=w520:dbl[], "System Preset.Test Configuration.Z Up"=w509:dbl, "System Preset.Test Configuration.Z Up 2"=w508:dbl)
            n163 = Send Notification(notification=w520, notifier=w532) -> ()  [unwired: 1 in, 2 out]
            n164 = call-poly "Name to ref convert.vi"("name"="Alarm Log") -> ("First REF"=w523:refnum<vi>)  [unwired: 10 in]
            n165 = for {
              tunnel: string[] ["X%0.1f ", "Y%0.1f "] ("format string") -> [w542] mode=indexing
              tunnel: w520 -> [w541] mode=indexing
              shift-right: [w540] -> w517
              shift-left: "" -> [w539]
              n166 = Format Into String(format string=w542, initial string=w539, w541) -> (resulting string=w540:string)  [unwired: 1 in, 1 out]
            }
            n167 = Build Array (concatenate)(w520, w509, w508) -> (w506:dbl[])
            n168 = Bundle By Name(cluster=T10 {"Wait"=0.0, "Next Step"="", "Writer Queue"=refnum, "Reset"=FALSE, "Target"=[]} ("s? t:f"), "Wait"=w514, "Target"=w506) -> (w510:T10)
            n169 = Type Cast(type=refnum<vi> refnum ("LOG"), x=w523) -> (*(type *) &x=w525:refnum<vi>)
            n170 = call-poly "Enqueue Message.vi"("Message Data"=w510, "Message"="Update Settings", "Message Queue"=w531) -> ("dup Message Queue"=w507:refnum<queue>)  [unwired: 7 in, 1 out]
            n171 = Format Into String(format string="Movement to %s has started", w517) -> (resulting string=w515:string)  [unwired: 2 in, 1 out]
            n172 = call-poly "Enqueue Message.vi"("Message Data"=w525, "Message"="Connect", "Message Queue"=w522) -> ()  [unwired: 7 in, 2 out]
            n173 = call-poly "Enqueue Message.vi"("Message Data"=w506, "Message"="Start", "Message Queue"=w507) -> ()  [unwired: 7 in, 2 out]
            n174 = Bundle By Name(cluster=cluster{"Replace":bool, "String":string} {"Replace"=FALSE, "String"="Procedure was started"}, "String"=w515) -> (w529:cluster{"Replace":bool, "String":string})
            n175 = call-poly "Enqueue Message.vi"("Message Data"=w529, "Message"="Update" ("Main CMD"), "Message Queue"=w528) -> ()  [unwired: 7 in, 2 out]
            n176 = Bundle By Name(cluster=w533, "Ready"=bool[] [FALSE, FALSE]) -> (w536:T4)
          }
          frame "Stop" {
            # "Start - Configure and start the acquisition."
            n177 = Flush Queue(queue=w574) -> ()  [unwired: 1 in, 3 out]
            n178 = Unbundle By Name(w551) -> ("Current SP"=w550:dbl[], "System Preset.Test Configuration.Z Up"=w549:dbl)  [unwired: 1 out]
            n179 = Unbundle By Name(w560) -> ("MOTOR"=w555:refnum<queue>, "MOTION"=w559:refnum<queue>)
            n180 = Unbundle By Name(w560) -> ("LOG"=w561:refnum<queue>)
            n181 = Build Array (concatenate)(w550, w549, 0.0 ("element")) -> (w547:dbl[])
            n182 = call "AM Stop.vi"("Message Queues out"=w560, "Data Cluster"=w551) -> ("error out"=w570:errorcluster)  [unwired: 8 in, 1 out]
            n183 = call-poly "Enqueue Message.vi"("Priority Message? (F)"=TRUE, "Message"="Stop", "Message Queue"=w559) -> ("error out"=w556:errorcluster)  [unwired: 7 in, 1 out]
            n184 = call "Send to Home.vi"("from local"=FALSE, "error in (no error)"=w556, "position"=w547, "Mototr Queue in"=w555) -> ("error out"=w546:errorcluster)  [unwired: 6 in, 1 out]
            n185 = call "Send to Home.vi"("from local"=TRUE, "error in (no error)"=w546) -> ("error out"=w545:errorcluster)  [unwired: 8 in, 1 out]
            n186 = Merge Errors(w570, w545) -> (w567:errorcluster)
            n187 = Format Into String(format string="%s has finished", Test_Type."Test" ("Test Type")) -> (resulting string=w562:string)  [unwired: 2 in, 1 out]
            n188 = Bundle By Name(cluster=w551, "Ready"=bool[] [FALSE, FALSE]) -> (w571:T4)
            n189 = Bundle By Name(cluster=cluster{"Replace":bool, "String":string} {"Replace"=FALSE, "String"="Procedure was started"}, "String"=w562) -> (w563:cluster{"Replace":bool, "String":string})
            n190 = call "Popup Dialog CLBK.vi"("error in"=w567, "Delay (5sec)"=-1.0, "Tab Control"=Popup_Dialog_States."Complete") -> ()  [unwired: 6 in, 3 out]
            n191 = call "FGV On Motion.vi"("CMD"=PCT_FGV_CMD."SET", "input"=FALSE) -> ()  [unwired: 8 in, 2 out]
            n192 = call-poly "Enqueue Message.vi"("Message Data"=w563, "Message"="Update" ("Main CMD"), "Message Queue"=w561) -> ()  [unwired: 7 in, 2 out]
          }
          frame "Abort" {
            w578 = "Test"  # String
            w587 = TRUE ("Priority Message? (F)")
            # "Start - Configure and start the acquisition."
            n193 = Unbundle By Name(w591) -> ("LOG"=w592:refnum<queue>, "MOTOR"=w586:refnum<queue>)
            n194 = call "FGV On Motion.vi"("CMD"=PCT_FGV_CMD."SET", "input"=FALSE) -> ()  [unwired: 8 in, 2 out]
            n195 = Unbundle By Name(w591) -> ("Procedure"=w600:refnum<queue>, "MOTION"=w589:refnum<queue>)
            n196 = Flush Queue(queue=w603) -> ()  [unwired: 1 in, 3 out]
            n197 = Unbundle By Name(w590) -> ()  [unwired: 1 out]
            n198 = call-poly "Enqueue Message.vi"("Priority Message? (F)"=w587, "Message"="Abort", "Message Queue"=w600) -> ()  [unwired: 7 in, 2 out]
            n199 = call-poly "Enqueue Message.vi"("Priority Message? (F)"=w587, "Message"="Stop", "Message Queue"=w589) -> ("error out"=w585:errorcluster)  [unwired: 7 in, 1 out]
            n200 = disable-structure shown="Enabled" {
              disable-tunnel: w586 -> [w606 _]
              disable-tunnel: w585 -> [w605 _]
              frame Disabled {
                n201 = call "Send to Home.vi"("error in (no error)"=w605, "Mototr Queue in"=w606) -> ()  [unwired: 8 in, 2 out]
              }
              frame Enabled {
              }
            }
            n202 = Format Into String(format string="%s has Aborted", Test_Type."Test" ("Test Type")) -> (resulting string=w593:string)  [unwired: 2 in, 1 out]
            n203 = Bundle By Name(cluster=w590, "Ready"=bool[] [FALSE, FALSE]) -> (w599:T4)
            n204 = call-poly "Enqueue Message.vi"("Message Data"=TRUE, "Message"="Stop", "Message Queue"=w582) -> ()  [unwired: 7 in, 2 out]
            n205 = Bundle By Name(cluster=cluster{"Replace":bool, "String":string} {"Replace"=FALSE, "String"="Procedure was started"}, "String"=w593) -> (w594:cluster{"Replace":bool, "String":string})
            n206 = call-poly "Enqueue Message.vi"("Message Data"=w594, "Message"="Update" ("Main CMD"), "Message Queue"=w592) -> ("dup Message Queue"=w577:refnum<queue>)  [unwired: 7 in, 1 out]
            n207 = call-poly "Enqueue Message.vi"("Message Data"=w578, "Message"="Save" ("Main CMD"), "Message Queue"=w577) -> ()  [unwired: 7 in, 2 out]
          }
          frame "Disconnect" {
            # "Start - Configure and start the acquisition."
            n208 = Flush Queue(queue=w608) -> ()  [unwired: 1 in, 3 out]
          }
          frame "Save" {
            # "Start - Configure and start the acquisition."
            n209 = call "AM Save.vi"("error in (no error)"=w616, "Message Data"=w614, "Message Queues out"=w613, "Data Cluster"=w617) -> ("error out"=w615:errorcluster, "Data Cluster out"=w618:T4)  [unwired: 6 in]
            n210 = call-poly "Enqueue Message.vi"("Message"="Temperature CW", "Message Queue"=w612) -> ()  [unwired: 8 in, 2 out]
          }
          frame "Send Response" {
            # "Acquire - Acquire data from the hardware. Since this is a continuous acquisition, this message will always message itself to run again."
            n211 = Unbundle By Name(w621) -> ("Writer Queue"=w620:refnum<queue>)
            n212 = call-poly "Enqueue Message.vi"("error in (no error)"=w624, "Message Data"=w622, "Message"="LOG Response", "Message Queue"=w620) -> ("error out"=w623:errorcluster)  [unwired: 6 in, 1 out]
          }
          frame "Update Settings" {
            # "New settings are available, update the current ones stored in the shift register with the settings sent as part of the message"
            n213 = Variant To Data(error in=w628, type=w630, Variant=w633) -> (data=w631:T4, error out=w632:errorcluster)
            n214 = Merge Errors(w628) -> (w634:errorcluster)
            n215 = Select(t=w630, s=w632, f=w631) -> (s? t:f=w629:T4)
          }
          frame "Exit" {
            # "Stop the VI"
            # "Exit - Send the Exit message to the UI Message Handler."
            n216 = Release Queue(queue=w636, error in (no error)=w638) -> (error out=w637:errorcluster)  [unwired: 1 in, 2 out]
            n217 = Merge Errors(w637) -> (w640:errorcluster)
          }
          frame Default {
            # "'Default' case only runs if there is a message that isn't defined in any of the other cases.  Output a programming error."
            n218 = xnode "Error Ring"("parameter 0"=w642) -> ("error out"=w643:errorcluster)
          }
        }
        n219 = disable-structure shown="Enabled" {
          disable-tunnel: [w49 _] -> w36
          disable-tunnel: w35 -> [w48 _]
          disable-tunnel: _ -> [w47 _]
          frame Disabled {
            n220 = call "Error Handler - Acquisition Message Loop.vi"("error in (no error)"=w48, "Message Queue"=w47) -> ("dup error in"=w49:errorcluster)  [unwired: 8 in, 1 out]
          }
          frame Enabled {
          }
        }
      }
    }
    frame Error {
    }
  }
  "error out" <- w7
